vi "LVIS_UpdateTest.vi"(8 "Error In":errorcluster, 11 "TestName":string) -> (0 "Error out":errorcluster, 3 "TestInfo":T1)   [LabVIEW 2015]
doc: "Updates the Test info based on the LVIS_Settings file configuration values."
uses:
  Globals/LVIS_IsGlobal.vi
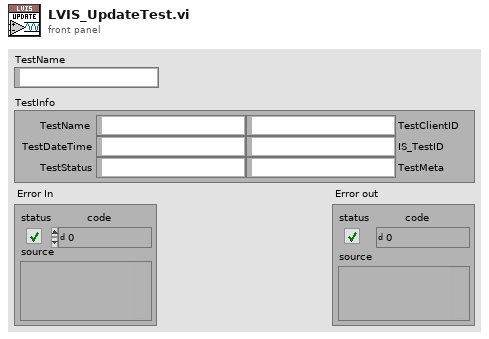
[diagram p1: front panel]
types:
  T1 = cluster{"TestName":string, "TestDateTime":string, "TestStatus":string, "TestClientID":string, "IS_TestID":string, "TestMeta":string}
  T2 = cluster{"[0]":string, "[1]":string, "[2]":string, "[3]":string, "[4]":string, "[5]":string}
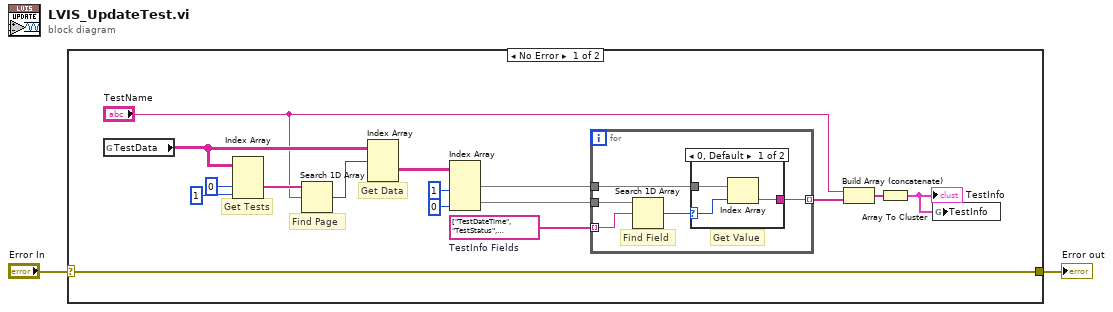
[diagram p0: block diagram]
diagram:
  n1 = case shown="No Error" "Error In" {
    selector: "Error In" -> [w9 w27]
    tunnel: [w9 w27] -> w1
    frame No Error {
      w10 = string[] ["TestDateTime", "TestStatus", "TestClientID", "IS_TestID", "TestMeta"]  # TestInfo Fields
      # "Get Data"
      # "Find Page"
      # "Get Tests"
      n2 = global read "LVIS_IsGlobal.vi" "TestData"() -> (w16:string[][][])
      n3 = Index Array(array=w16, index (dim 1)=0 ("disabled index (row)"), index (dim 2)=1 ("disabled index (col)")) -> (element=w17:string[])  [unwired: 1 in]
      n4 = Search 1D Array(1D array=w17, element="TestName") -> (index of element=w15:i32)  [unwired: 1 in]
      n5 = Index Array(array=w16, index (dim 0)=w15) -> (element=w5:string[][])  [unwired: 2 in]
      n6 = Index Array(array=w5, index (col) #1=1 ("disabled index (col)"), index (col) #2=0 ("index (col)")) -> (element #1=w12:string[], element #2=w11:string[])  [unwired: 2 in]
      n7 = for {
        tunnel: w12 -> [w20]
        tunnel: w11 -> [w23]
        tunnel: w10 -> [w22] mode=indexing
        tunnel: [w19] -> w8 mode=indexing
        # "Get Value"
        # "Find Field"
        n8 = Search 1D Array(1D array=w23, element=w22) -> (index of element=w21:i32)  [unwired: 1 in]
        n9 = case shown="0, Default" w21 {
          selector: w21 -> [w25 _]
          tunnel: w20 -> [w26 _]
          tunnel: [w24 _] -> w19
          frame 0, Default {
            n10 = Index Array(array=w26, index=w25) -> (element=w24:string)
          }
          frame -1 {
            # "Blank if\nnot found"
          }
        }
      }
      n11 = Build Array (concatenate)("TestName", w8) -> (w6:string[])
      n12 = Array To Cluster(array=w6) -> (cluster=w4:T2)
      "TestInfo" <- w4
      n13 = global write "LVIS_IsGlobal.vi" "TestInfo"(w4) -> ()
    }
    frame Error {
    }
  }
  "Error out" <- w1
